vi "Labview.vi"() -> ()   [LabVIEW 2017]
uses:
  <vilib>/Utility/inputDevices.llb/joystickAcquire.vi
  <vilib>/Platform/NI_3dgraph.lvlib
panel:
  in  "S1":dbl
  in  "S2":dbl
  in  "3D Curve":refnum<k7>(container)
  out "L6":dbl(slide) scale=0.35..0.65
  out "L5":dbl(slide) scale=0.35..0.65
  out "L4":dbl(slide) scale=0.35..0.65
  out "L3":dbl(slide) scale=0.35..0.65
  out "L2":dbl(slide) scale=0.35..0.65
  out "L1":dbl(slide) scale=0.35..0.65
  in  "error in (no error)":errorcluster
  out "K2":dbl
  out "Phi2":dbl
  out "K1":dbl
  out "Phi1":dbl
  in  "rate":dbl
  out "Numeric":dbl
  out "error out":errorcluster
  in  "stop":bool
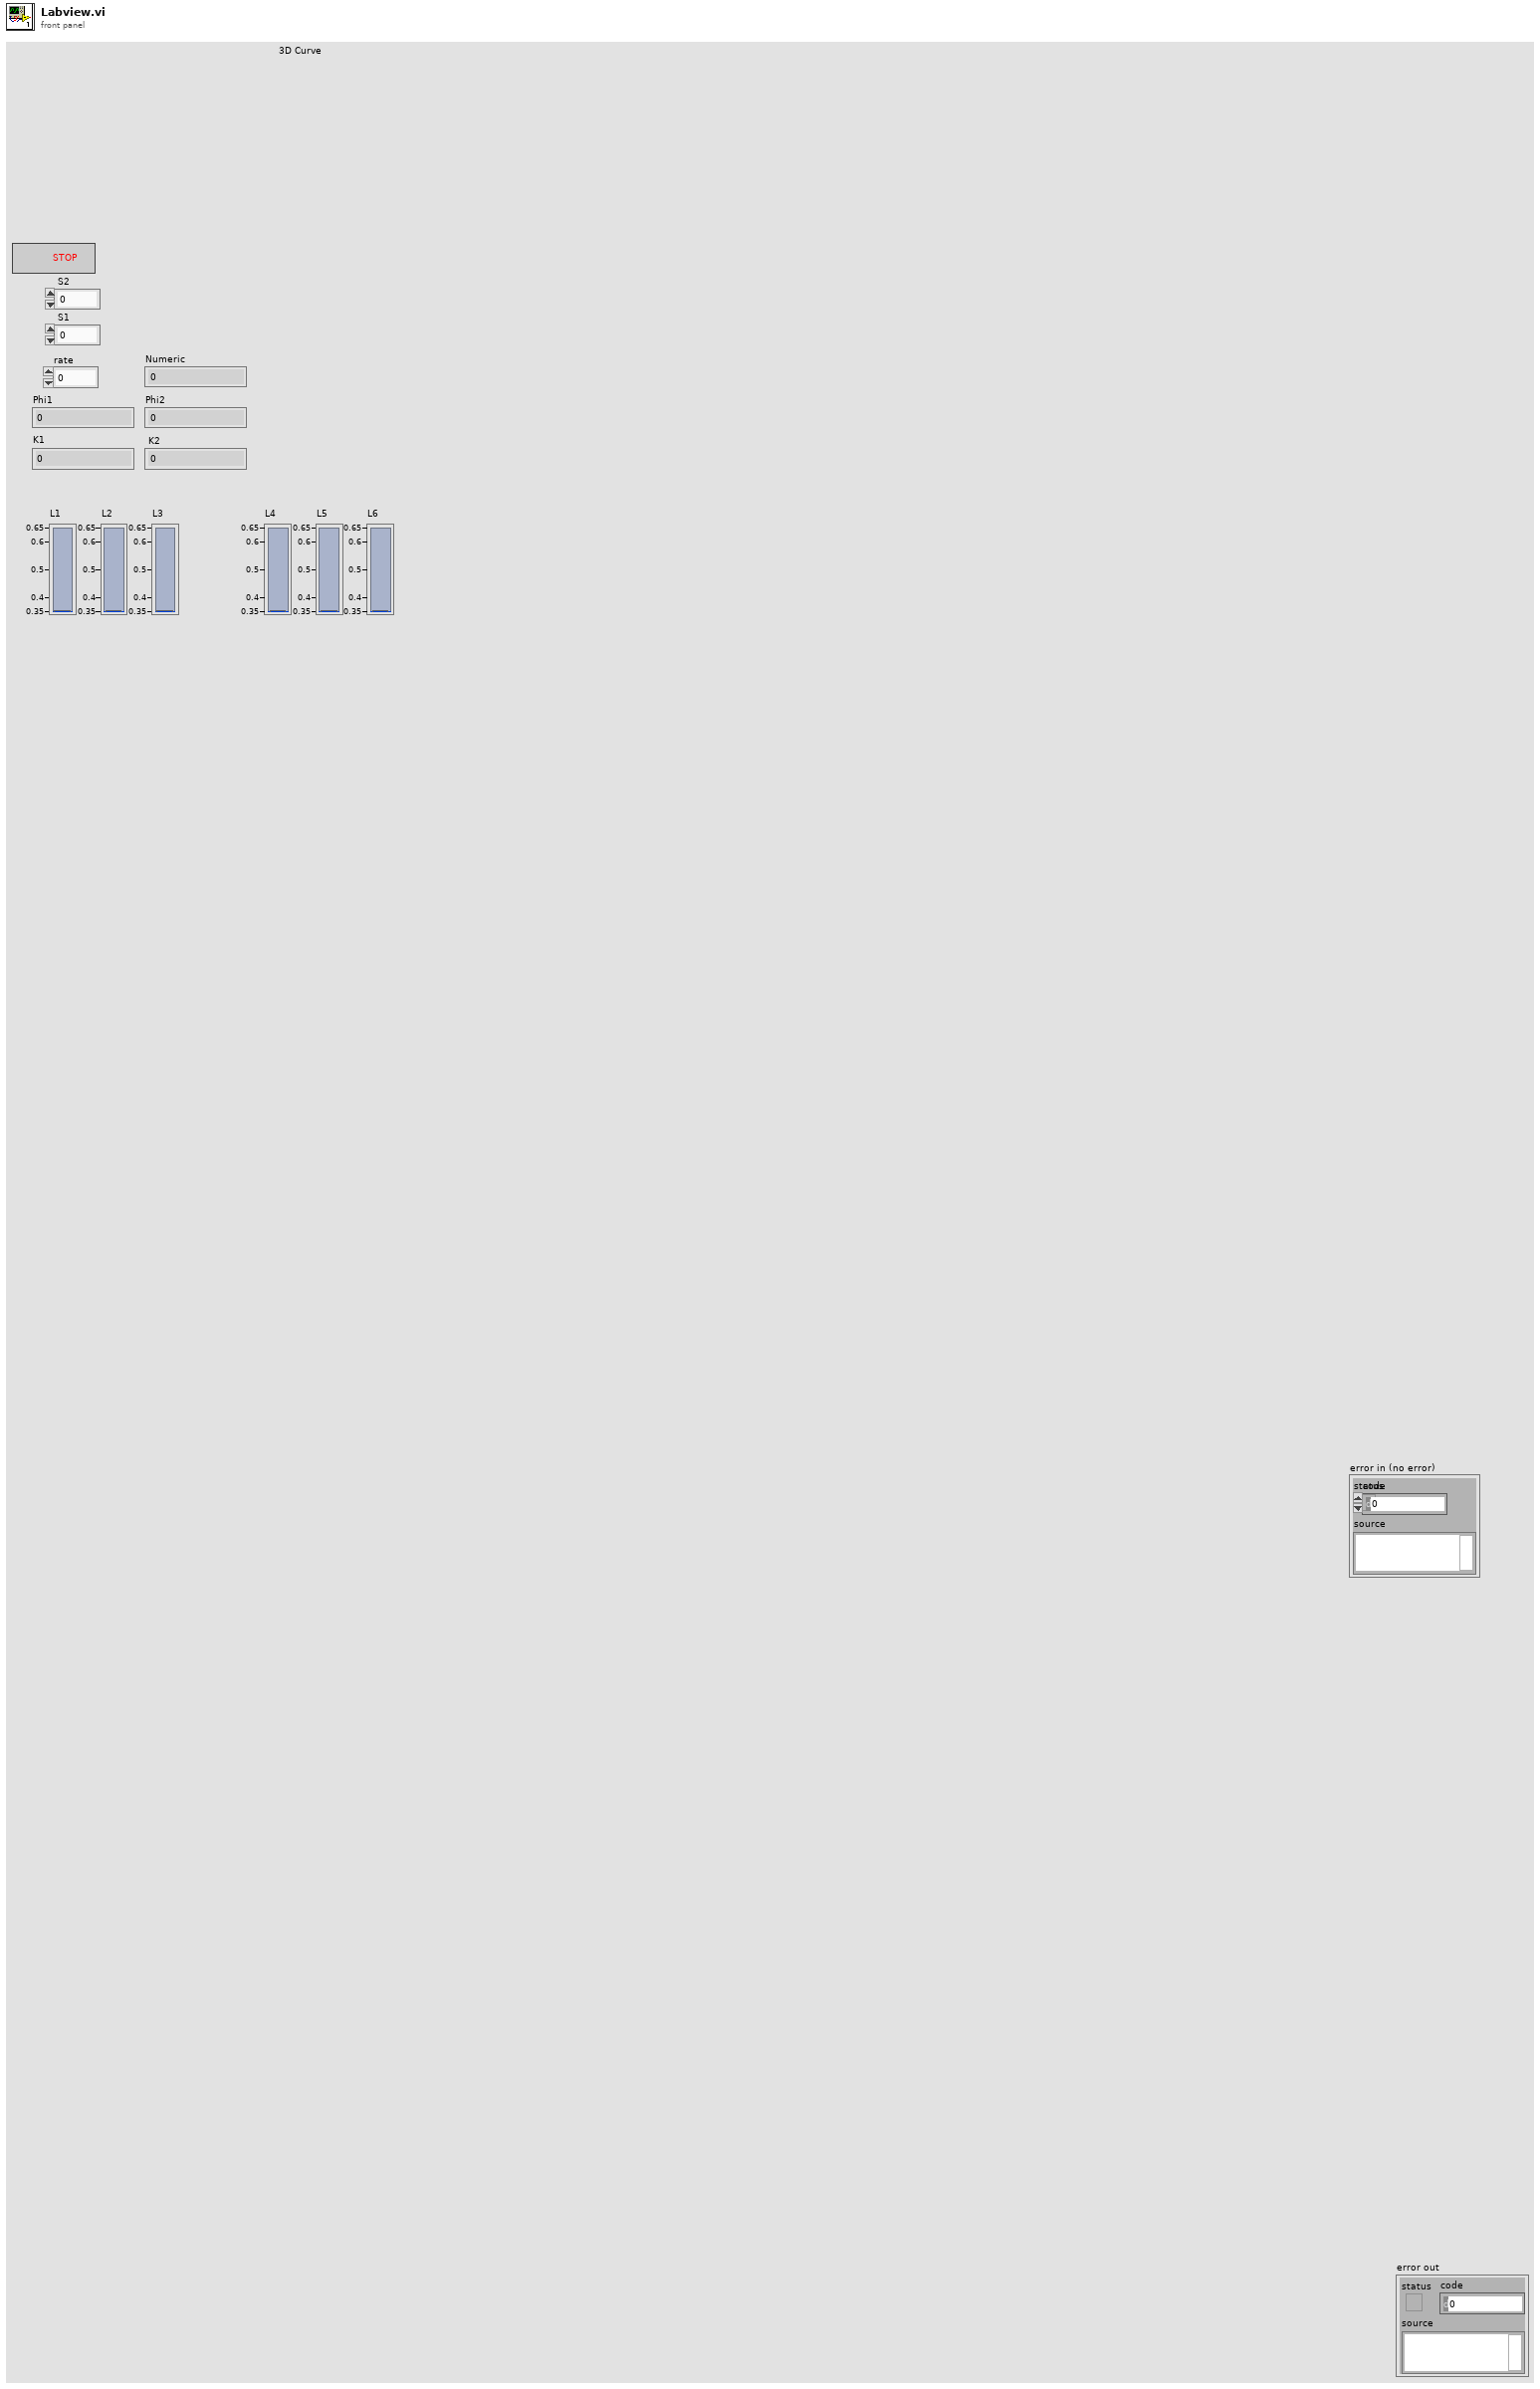
[diagram p1: front panel]
types:
  T1 = cluster{"X axis":i32, "Y axis":i32, "Z axis":i32, "X axis rotation":i32, "Y axis rotation":i32, "Z axis rotation":i32, "U axis":i32, "V axis":i32}
  T2 = cluster{"button 1":bool, "button 2":bool, "button 3":bool, "button 4":bool, "button 5":bool, "button 6":bool, "button 7":bool, "button 8":bool, "button 9":bool, "button 10":bool, "button 11":bool, "button 12":bool, "button 13":bool, "button 14":bool, "button 15":bool, "button 16":bool, "button 17":bool, "button 18":bool, "button 19":bool, "button 20":bool, "button 21":bool, "button 22":bool, "button 23":bool, "button 24":bool, "button 25":bool, "button 26":bool, "button 27":bool, "button 28":bool, "button 29":bool, "button 30":bool, "button 31":bool, "button 32":bool}
  T3 = cluster{"pov 1":i32, "pov 2":i32, "pov 3":i32, "pov 4":i32}
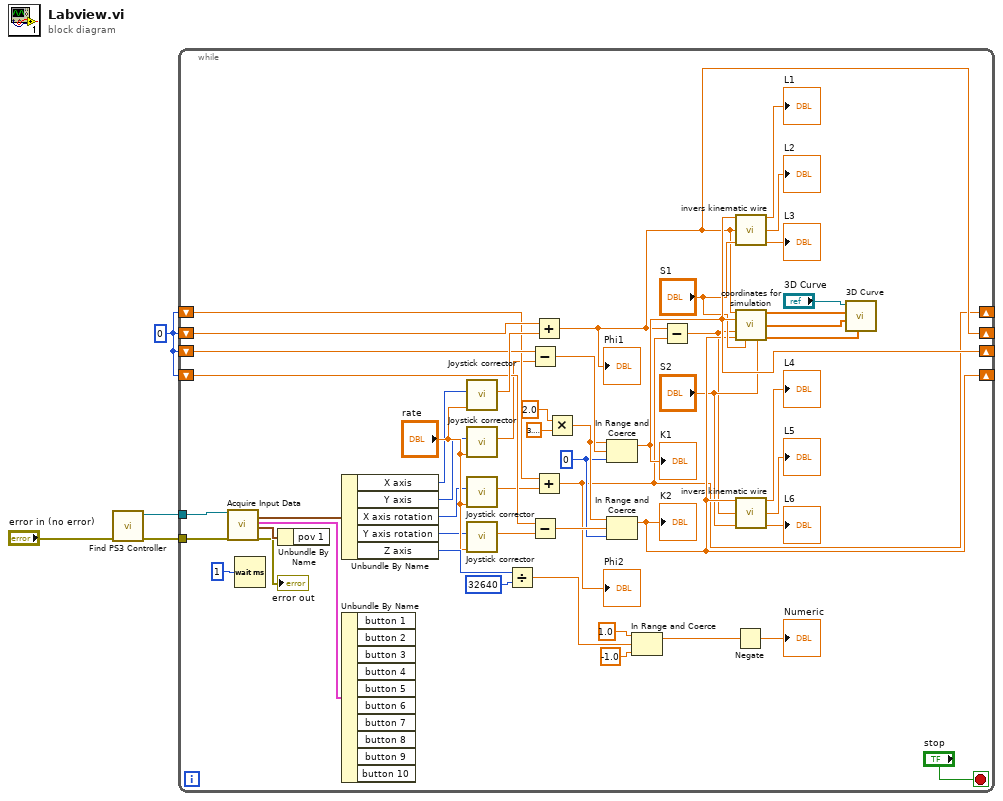
[diagram p0: block diagram]
diagram:
  w2 = 0
  n1 = call "Find PS3 Controller.vi"("error in (no error)"="error in (no error)") -> ("error out"=w4:errorcluster, "Controller Reference Out"=w3:refnum<k1>)  [unwired: 9 in]
  n2 = while {
    tunnel: w4 -> [w48]
    tunnel: w3 -> [w49]
    shift-right: [w7] -> _
    shift-left: w2 -> [w35]
    shift-right: [w12] -> _
    shift-left: w2 -> [w31]
    shift-right: [w6] -> _
    shift-left: w2 -> [w30]
    shift-right: [w10] -> _
    shift-left: w2 -> [w29]
    stop <- "stop" stop-if-true
    w22 = 0
    n3 = call-poly <vilib>:"Acquire Input Data.vi"("device ID"=w49, "error in (no error)"=w48) -> ("axis info"=w50:T1, "button info"=w53:T2, "direction info"=w52:T3, "error out"=→"error out":errorcluster)  [unwired: 14 out]
    n4 = Wait (ms)(milliseconds to wait=u32 1) -> ()  [unwired: 1 out]
    n5 = Unbundle By Name(w52) -> ()  [unwired: 1 out]
    n6 = Unbundle By Name(w50) -> ("X axis"=w36:i32, "Y axis"=w37:i32, "X axis rotation"=w38:i32, "Y axis rotation"=w39:i32, "Z axis"=w46:i32)
    n7 = Unbundle By Name(w53) -> ()  [unwired: 10 out]
    n8 = call "Joystick corrector.vi"("rate"="rate", "Joystick"=w36) -> ("output"=w34:dbl)  [unwired: 9 in]
    n9 = call "Joystick corrector.vi"("rate"="rate", "Joystick"=w37) -> ("output"=w26:dbl)  [unwired: 9 in]
    n10 = call "Joystick corrector.vi"("rate"="rate", "Joystick"=w38) -> ("output"=w27:dbl)  [unwired: 9 in]
    n11 = call "Joystick corrector.vi"("rate"="rate", "Joystick"=w39) -> ("output"=w28:dbl)  [unwired: 9 in]
    n12 = Divide(x=w46, y=32640) -> (x/y=w43:dbl)
    n13 = Subtract(x=w31, y=w26) -> (x-y=w25:dbl)
    n14 = Subtract(x=w29, y=w28) -> (x-y=w24:dbl)
    n15 = Add(x=w35, y=w34) -> (x+y=w7:dbl)
    "Phi1" <- w7
    n16 = Add(x=w30, y=w27) -> (x+y=w6:dbl)
    "Phi2" <- w6
    n17 = Multiply(x=2.0 ("upper limit"), y=3.141592653589793) -> (x*y=w23:dbl)
    n18 = In Range and Coerce(upper limit=w23, x=w25, lower limit=w22) -> (coerced(x)=w12:dbl)  [unwired: 1 out]
    "K1" <- w12
    n19 = In Range and Coerce(upper limit=w23, x=w24, lower limit=w22) -> (coerced(x)=w10:dbl)  [unwired: 1 out]
    "K2" <- w10
    n20 = In Range and Coerce(upper limit=1.0, x=w43, lower limit=-1.0) -> (coerced(x)=w42:dbl)  [unwired: 1 out]
    n21 = Subtract(x=w7, y=w6) -> (x-y=w5:dbl)
    n22 = Negate(x=w42) -> (-x=→"Numeric":dbl)
    n23 = call "invers kinematic wire.vi"("K"=w12, "phi"=w7, "s"="S1") -> ("L1"=→"L1":dbl, "L 2"=→"L2":dbl, "L 3"=→"L3":dbl)  [unwired: 10 in]
    n24 = call "coordinates for simulation.vi"("phi1"=w7, "k1"=w12, "phi2"=w5, "k2"=w10, "s1"="S1", "s2"="S2") -> ("X"=w15:dbl[], "Y"=w14:dbl[], "Z"=w13:dbl[])  [unwired: 7 in]
    n25 = call "invers kinematic wire.vi"("K"=w10, "phi"=w5, "s"="S2") -> ("L1"=→"L4":dbl, "L 2"=→"L5":dbl, "L 3"=→"L6":dbl)  [unwired: 10 in]
    n26 = call <vilib>:"3D Curve.vi"("z vector"=w13, "y vector"=w14, "x vector"=w15, "3D graph"="3D Curve") -> ()  [unwired: 6 in, 2 out]
  }
